vi "Untitled 4.vi"() -> ()   [LabVIEW 2015]
uses:
  Drive Metrics.ctl
  Drive States.ctl
  Copilot States.ctl
panel:
  in  "Drive Metrics":T1
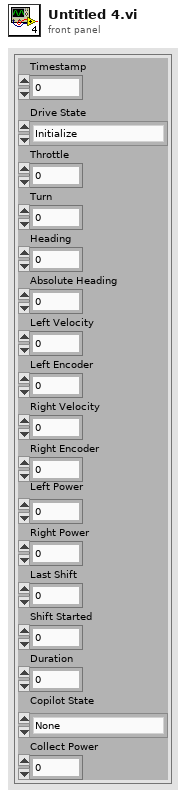
[diagram p1: front panel]
types:
  T1 = typedef "Drive Metrics.ctl" = cluster{"Timestamp":u32, "Drive State":T2, "Throttle":dbl, "Turn":dbl, "Heading":dbl, "Absolute Heading":dbl, "Left Velocity":dbl, "Left Encoder":dbl, "Right Velocity":dbl, "Right Encoder":dbl, "Left Power":dbl, "Right Power":dbl, "Last Shift":u32, "Shift Started":u32, "Duration":i64, "Copilot State":T3, "Collect Power":dbl}
  T2 = typedef "Drive States.ctl" = enum16{"Initialize", "Low Gear", "Up Shift Begin", "Up Shifting", "Up Shift Delay", "High Gear", "Down Shift Begin", "Down Shifting", "Down Shift Delay"}
  T3 = typedef "Copilot States.ctl" = enum16{"None", "Collect", "Eject"}
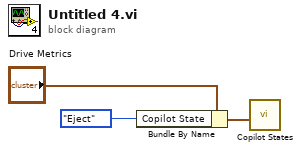
[diagram p0: block diagram]
diagram:
  n1 = Bundle By Name(cluster="Drive Metrics", "Copilot State"=Copilot_States."Eject") -> (w2:T1)
  n2 = call "Copilot States.vi"("Drive Metrics in"=w2) -> ()  [unwired: 10 in, 1 out]
